vi "Publish Measurement Pin DBL.vi"(0 "TSM context in":T1, 1 "Published Data Id In":string, 5 "Measurement Data (row - per site)":dbl[][](array[numeric]), 7 "Expanded Pin List in":tag[](array[tag]), 11 "error in":errorcluster) -> (4 "TSM context out":T1, 6 "Published Data Id Out":string[](array[string]), 8 "Expanded Pin List out":tag[](array[tag]), 15 "error out":errorcluster)   [LabVIEW 2019]
doc: "The Measurement Data array input is expected to be in a per-site, per-pin format, where the rows represent the sites, and the columns represent the pins"
uses:
  <vilib>/NI_TestStand_SemiconductorModule/NI_TestStand_Semiconductor_Module.lvlibp/PinMap/General/SemiconductorModuleContext.ctl
  <vilib>/NI_TestStand_SemiconductorModule/NI_TestStand_Semiconductor_Module.lvlibp/PinMap/General/Publish/PublishDataDoubleFunctionalTest.vi
  <vilib>/NI_TestStand_SemiconductorModule/NI_TestStand_Semiconductor_Module.lvlibp
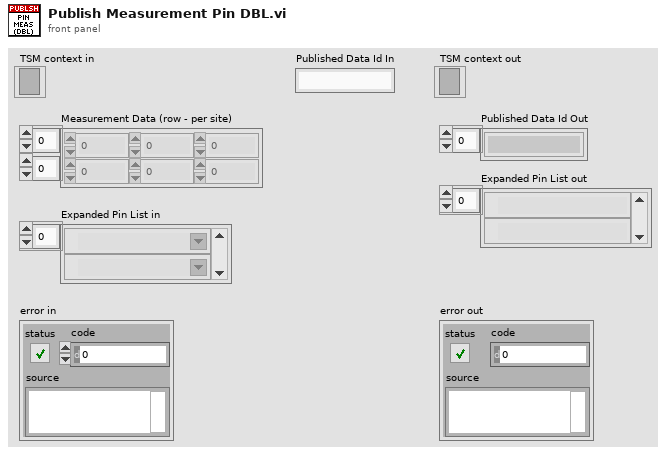
[diagram p1: front panel]
types:
  T1 = typedef "NI_TestStand_Semiconductor_Module.lvlibp/SemiconductorModuleContext.ctl" = refnum<k7>
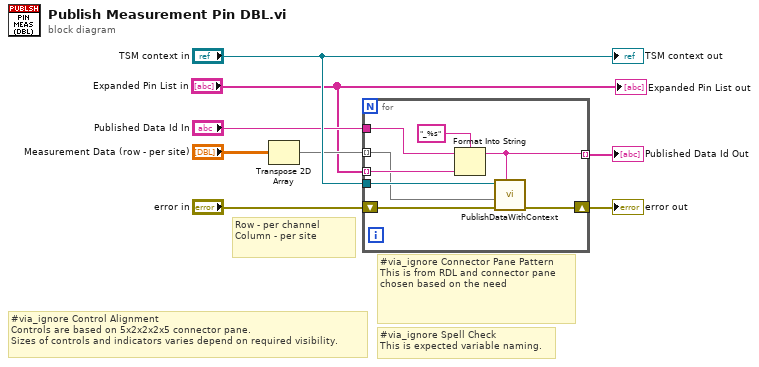
[diagram p0: block diagram]
diagram:
  # "#via_ignore Control Alignment\nControls are based on 5x2x2x2x5 connector pane.\nSizes of controls and indicators varies depend on required visibility."
  # "#via_ignore Spell Check\nThis is expected variable naming."
  # "Row - per channel\nColumn - per site"
  # "#via_ignore Connector Pane Pattern\nThis is from RDL and connector pane chosen based on the need"
  n1 = Transpose 2D Array(2D array="Measurement Data (row - per site)") -> (transposed array=w2:dbl[][])
  n2 = for {
    tunnel: "TSM context in" -> [w16]
    tunnel: w2 -> [w10] mode=indexing
    shift-right: [w12] -> w6
    shift-left: "error in" -> [w15]
    tunnel: "Expanded Pin List in" -> [w13] mode=indexing
    tunnel: "Published Data Id In" -> [w11]
    tunnel: [w9] -> w3 mode=indexing
    n3 = Format Into String(format string="_%s", initial string=w11, w13) -> (resulting string=w9:string)  [unwired: 1 in, 1 out]
    n4 = call-poly <vilib>:"PublishDataWithContext.vi"("Published Data Id"=w9, "error in (no error)"=w15, "Data In"=w10, "Semiconductor Module Context"=w16) -> ("error out"=w12:errorcluster)  [unwired: 6 in, 1 out]
  }
  "error out" <- w6
  "Published Data Id Out" <- w3
  "TSM context out" <- "TSM context in"
  "Expanded Pin List out" <- "Expanded Pin List in"
